vi "Load Macro.vi"(7 "Macro Name":string, 8 "error in (no error)":errorcluster, 11 "refnum":T5) -> (0 "error out":errorcluster, 2 "Macro":T1, 3 "refnum out":T5)   [LabVIEW 2020, in "MacroAssert.lvlib"]
doc: "Loads the macro defined by <B>Macro Name</B> from the config file defined by <B>refnum</B>."
uses:
  MacroAssert.lvlib
  <vilib>/Utility/config.llb/Config Data RefNum.ctl
  CTLs/Macro Cluster V3.ctl
  CTLs/Macro Config V3.ctl
  CTLs/Step V3.ctl
  CTLs/Step Type V3.ctl
  CTLs/Macro Cluster V1.ctl
  CTLs/Step V1-2.ctl
  CTLs/Step Type V1-2.ctl
  CTLs/Macro Cluster V2.ctl
  <vilib>/Utility/config.llb/Read Key (String).vi
  <vilib>/Utility/config.llb/Read Key (U32).vi
  <vilib>/Utility/config.llb/Read Key (I32).vi
  <vilib>/Utility/error.llb/Error Cluster From Error Code.vi
  <vilib>/ErrorRing/Error Ring.xnode
  <vilib>/Utility/config.llb/NI_LVConfig.lvlib
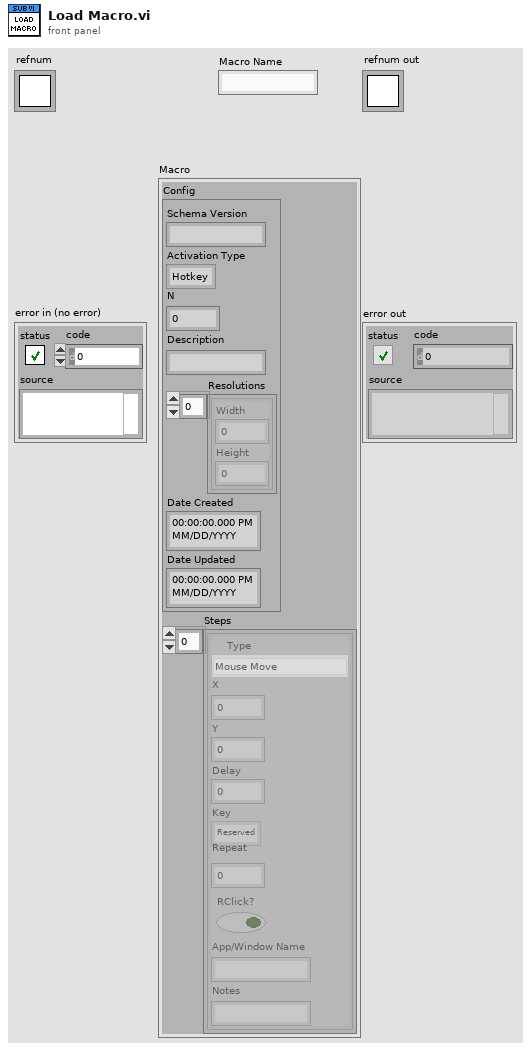
[diagram p1: front panel]
types:
  T1 = typedef "MacroAssert.lvlib/Macro Cluster V3.ctl" = cluster{"Config":T2, "Steps":T3[]}
  T2 = typedef "MacroAssert.lvlib/Macro Config V3.ctl" = cluster{"Schema Version":string, "Activation Type":enum32{"Hotkey", "Automatic"}, "N":i32, "Description":string, "Resolutions":cluster{"Width":i16, "Height":i16}[], "Date Created":timestamp, "Date Updated":timestamp}
  T3 = typedef "MacroAssert.lvlib/Step V3.ctl" = cluster{"Type":T4, "X":i32, "Y":i32, "Delay":i32, "Key":u8, "Repeat":i32, "RClick?":bool, "App/Window Name":string, "Notes":string}
  T4 = typedef "MacroAssert.lvlib/Step Type V3.ctl" = enum16{"Mouse Move", "Mouse Click", "Key Press", "Wait", "Mouse Down", "Mouse Up", "Key Down", "Key Up", "Run Application", "Maximize Window", "Restore Window", "Minimize Window", "Close Window", "Bring Window to Front", "Send Window to Back"}
  T5 = typedef "NI_LVConfig.lvlib/Config Data RefNum.ctl" = refnum<k1>
  T6 = typedef "MacroAssert.lvlib/Macro Cluster V1.ctl" = cluster{"Steps":T7[], "Activation Type":enum32{"Hotkey", "Automatic"}, "N":i32}
  T7 = typedef "MacroAssert.lvlib/Step V1-2.ctl" = cluster{"Type":T8, "Coords":cluster{"x":i32, "y":i32}, "Delay":i32, "Key":u8, "Repeat":i32, "RClick?":bool}
  T8 = typedef "MacroAssert.lvlib/Step Type V1-2.ctl" = enum16{"Mouse Move", "Mouse Click", "Key Press", "Wait", "Mouse Down", "Mouse Up", "Key Down", "Key Up"}
  T9 = typedef "MacroAssert.lvlib/Macro Cluster V2.ctl" = cluster{"Steps":T7[], "Activation Type":enum32{"Hotkey", "Automatic"}, "N":i32, "Description":string, "Resolutions":cluster{"Width":i16, "Height":i16}[], "Date Created":timestamp, "Date Updated":timestamp}
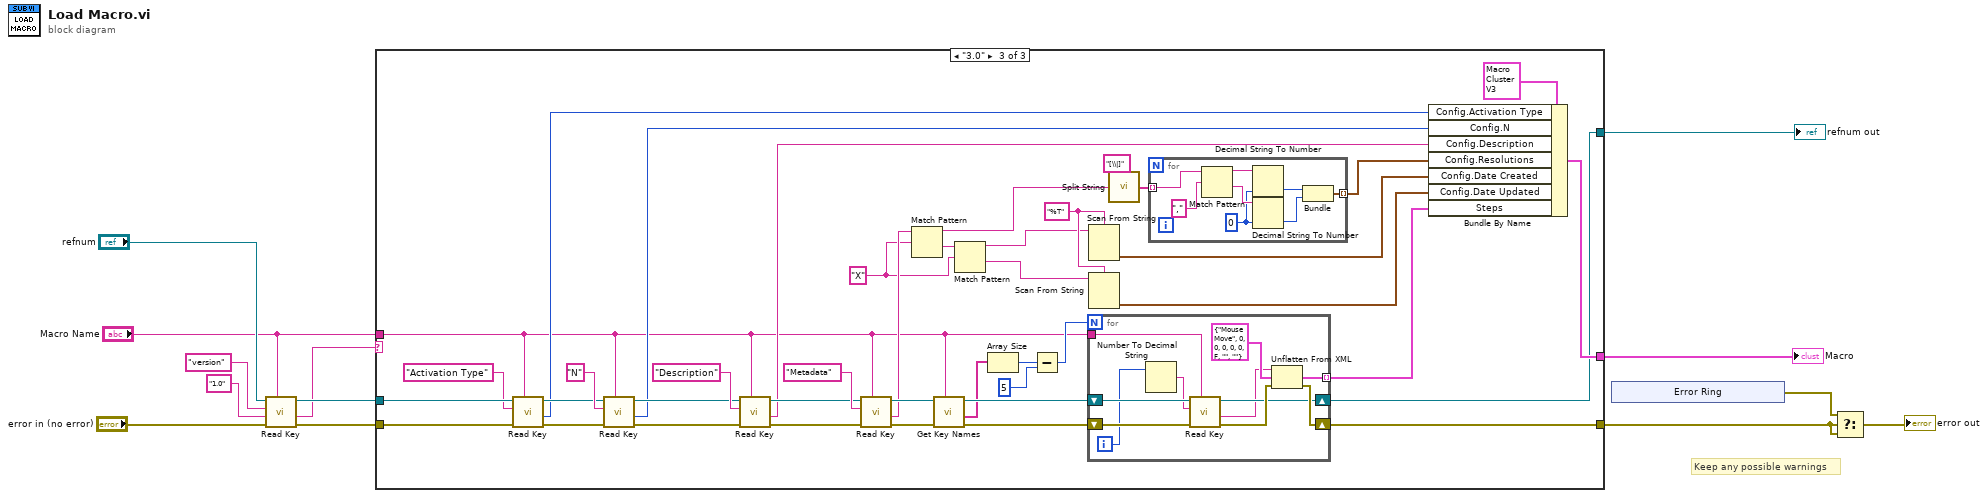
[diagram p0: block diagram]
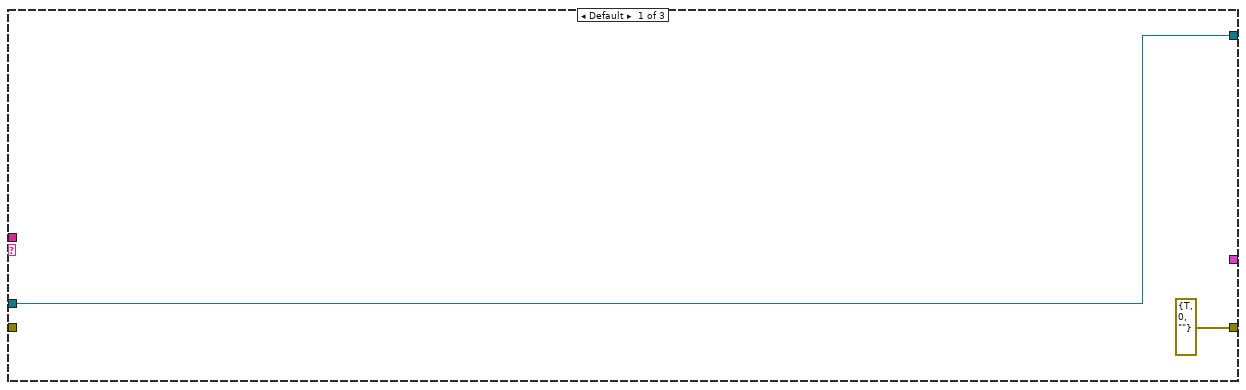
[diagram p2: hidden frame]
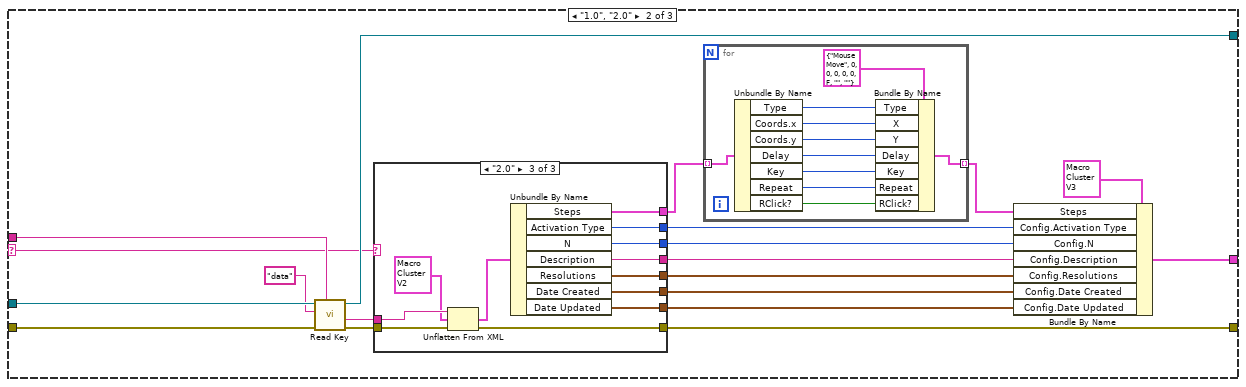
[diagram p3: hidden frame]
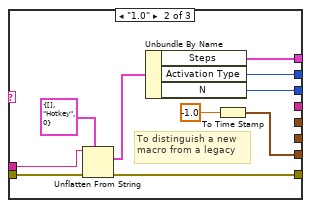
[diagram p5: hidden frame]
diagram:
  # "Keep any possible warnings"
  n1 = call-poly <vilib>:"Read Key.vi"("section"="Macro Name", "error in (no error)"="error in (no error)", "default value"="1.0", "key"="version", "refnum"="refnum") -> ("error out"=w9:errorcluster, "value"=w5:string, "refnum out"=w12:T5)  [unwired: 3 in, 1 out]
  n2 = case shown="\"3.0\"" w5 {
    selector: w5 -> [_ w27 _]
    tunnel: w12 -> [w15 w34 w108]
    tunnel: [w15 w30 w75] -> w11
    tunnel: w9 -> [_ w29 w106]
    tunnel: "Macro Name" -> [_ w28 w68]
    tunnel: [errorcluster {"status"=TRUE, "code"=0, "source"=""} ("error out") w20 w88] -> w3
    tunnel: [_ w19 w105] -> w4
    frame Default {
    }
    frame "1.0", "2.0" {
      n3 = call-poly <vilib>:"Read Key.vi"("section"=w28, "error in (no error)"=w29, "key"="data", "refnum"=w34) -> ("error out"=w31:errorcluster, "value"=w32:string, "refnum out"=w30:T5)  [unwired: 4 in, 1 out]
      n4 = case shown="\"2.0\"" w27 {
        tunnel: w32 -> [_ w55 w67]
        tunnel: w31 -> [w45 w54 w66]
        tunnel: [w45 w53 w65] -> w20
        tunnel: [_ w51 w63] -> w17
        tunnel: [_ w50 w62] -> w26
        tunnel: [_ w49 w61] -> w25
        tunnel: [_ _ w59] -> w24
        tunnel: [_ _ w58] -> w23
        tunnel: [_ _ w57] -> w22
        tunnel: [_ w46 w56] -> w21
        frame "False", Default {
        }
        frame "1.0" {
          # "To distinguish a new macro from a legacy"
          n5 = Unflatten From String(type=T6 {"Steps"=[], "Activation Type"=enum."Hotkey", "N"=0} ("Macro Cluster"), binary string=w55, error in (no error)=w54) -> (value=w52:T6, error out=w53:errorcluster)  [unwired: 2 in, 1 out]
          n6 = Unbundle By Name(w52) -> ("Steps"=w51:T7[], "Activation Type"=w50:enum32{"Hotkey", "Automatic"}, "N"=w49:i32)
          n7 = To Time Stamp(1:-1.0) -> (0:w46:timestamp)
        }
        frame "2.0" {
          n8 = Unflatten From XML(xml string=w67, type=T9 {"Steps"=[], "Activation Type"=enum."Hotkey", "N"=0, "Description"="", "Resolutions"=[], "Date Created"=timestamp(0 s since 1904-01-01), "Date Updated"=timestamp(0 s since 1904-01-01)} ("Macro Cluster"), error in (no error)=w66) -> (value=w64:T9, error out=w65:errorcluster)
          n9 = Unbundle By Name(w64) -> ("Steps"=w63:T7[], "Activation Type"=w62:enum32{"Hotkey", "Automatic"}, "N"=w61:i32, "Description"=w59:string, "Resolutions"=w58:cluster{"Width":i16, "Height":i16}[], "Date Created"=w57:timestamp, "Date Updated"=w56:timestamp)
        }
      }
      n10 = for {
        tunnel: w17 -> [w44] mode=indexing
        tunnel: [w37] -> w16 mode=indexing
        n11 = Unbundle By Name(w44) -> ("Type"=w36:T8, "Coords.x"=w42:i32, "Coords.y"=w35:i32, "Delay"=w41:i32, "Key"=w40:u8, "Repeat"=w39:i32, "RClick?"=w38:bool)
        n12 = Bundle By Name(cluster=T3 {"Type"=enum."Mouse Move", "X"=0, "Y"=0, "Delay"=0, "Key"=0, "Repeat"=0, "RClick?"=FALSE, "App/Window Name"="", "Notes"=""} ("Step"), "Type"=w36, "X"=w42, "Y"=w35, "Delay"=w41, "Key"=w40, "Repeat"=w39, "RClick?"=w38) -> (w37:T3)
      }
      n13 = Bundle By Name(cluster=T1 {"Config"={"Schema Version"="", "Activation Type"=enum."Hotkey", "N"=0, "Description"="", "Resolutions"=[], "Date Created"=timestamp(0 s since 1904-01-01), "Date Updated"=timestamp(0 s since 1904-01-01)}, "Steps"=[]} ("Macro Cluster"), "Steps"=w16, "Config.Activation Type"=w26, "Config.N"=w25, "Config.Description"=w24, "Config.Resolutions"=w23, "Config.Date Created"=w22, "Config.Date Updated"=w21) -> (w19:T1)
    }
    frame "3.0" {
      w72 = "X" ("Split Pattern")
      w91 = "%T" ("format string")
      n14 = call-poly <vilib>:"Read Key.vi"("section"=w68, "error in (no error)"=w106, "key"="Activation Type", "refnum"=w108) -> ("error out"=w101:errorcluster, "value"=w94:u32, "refnum out"=w102:T5)  [unwired: 4 in, 1 out]
      n15 = call-poly <vilib>:"Read Key.vi"("section"=w68, "error in (no error)"=w101, "key"="N", "refnum"=w102) -> ("error out"=w98:errorcluster, "value"=w93:i32, "refnum out"=w99:T5)  [unwired: 4 in, 1 out]
      n16 = call-poly <vilib>:"Read Key.vi"("section"=w68, "error in (no error)"=w98, "key"="Description", "refnum"=w99) -> ("error out"=w95:errorcluster, "value"=w92:string, "refnum out"=w96:T5)  [unwired: 4 in, 1 out]
      n17 = call-poly <vilib>:"Read Key.vi"("section"=w68, "error in (no error)"=w95, "key"="Metadata", "refnum"=w96) -> ("error out"=w83:errorcluster, "value"=w74:string, "refnum out"=w82:T5)  [unwired: 4 in, 1 out]
      n18 = Match Pattern(string=w74, regular expression=w72) -> (before substring=w71:string, after substring=w73:string)  [unwired: 1 in, 2 out]
      n19 = call <vilib>:"Get Key Names.vi"("section"=w68, "error in (no error)"=w83, "refnum"=w82) -> ("error out"=w81:errorcluster, "key names"=w79:string[], "refnum out"=w80:T5)  [unwired: 5 in, 1 out]
      n20 = Match Pattern(string=w73, regular expression=w72) -> (before substring=w70:string, after substring=w69:string)  [unwired: 1 in, 2 out]
      n21 = Array Size(array=w79) -> (size(s)=w78:i32)
      n22 = Subtract(x=w78, y=5) -> (x-y=w76:i32)
      n23 = for {
        N: w76 -> [_]
        tunnel: [w125] -> w87 mode=indexing
        shift-right: [w126] -> w88
        shift-left: w81 -> [w121]
        shift-right: [w122] -> w75
        shift-left: w80 -> [w124]
        tunnel: w68 -> [w120]
        i -> [w118]
        n24 = Number To Decimal String(number=w118) -> (decimal integer string=w119:string)  [unwired: 1 in]
        n25 = call-poly <vilib>:"Read Key.vi"("section"=w120, "error in (no error)"=w121, "key"=w119, "refnum"=w124) -> ("error out"=w123:errorcluster, "value"=w117:string, "refnum out"=w122:T5)  [unwired: 4 in, 1 out]
        n26 = Unflatten From XML(xml string=w117, type=T3 {"Type"=enum."Mouse Move", "X"=0, "Y"=0, "Delay"=0, "Key"=0, "Repeat"=0, "RClick?"=FALSE, "App/Window Name"="", "Notes"=""} ("Step"), error in (no error)=w123) -> (value=w125:T3, error out=w126:errorcluster)
      }
      n27 = Scan From String(format string=w91, input string=w70) -> (output 1=w90:timestamp)  [unwired: 3 in, 3 out]
      n28 = Scan From String(format string=w91, input string=w69) -> (output 1=w89:timestamp)  [unwired: 3 in, 3 out]
      n29 = call <vilib>:"Split String.vi"("Split Pattern"="[\\|]", "Input String"=w71) -> ("Split String"=w85:string[])  [unwired: 5 in]
      n30 = for {
        tunnel: w85 -> [w116] mode=indexing
        tunnel: [w110] -> w84 mode=indexing
        w109 = i16 0 ("default (0 I32)")
        n31 = Match Pattern(string=w116, regular expression=",") -> (before substring=w114:string, after substring=w113:string)  [unwired: 1 in, 2 out]
        n32 = Decimal String To Number(string=w114, default (0L)=w109) -> (number=w112:i16)  [unwired: 1 in, 1 out]
        n33 = Decimal String To Number(string=w113, default (0L)=w109) -> (number=w111:i16)  [unwired: 1 in, 1 out]
        n34 = Bundle(w112, w111) -> (w110:cluster{i16, i16})  [unwired: 1 in]
      }
      n35 = Bundle By Name(cluster=T1 {"Config"={"Schema Version"="", "Activation Type"=enum."Hotkey", "N"=0, "Description"="", "Resolutions"=[], "Date Created"=timestamp(0 s since 1904-01-01), "Date Updated"=timestamp(0 s since 1904-01-01)}, "Steps"=[]} ("Macro Cluster"), "Config.Activation Type"=w94, "Config.N"=w93, "Config.Description"=w92, "Config.Resolutions"=w84, "Config.Date Created"=w90, "Config.Date Updated"=w89, "Steps"=w87) -> (w105:T1)
    }
  }
  "refnum out" <- w11
  "Macro" <- w4
  n36 = xnode "Error Ring"() -> ("error out"=w2:errorcluster)
  n37 = Select(t=w2, s=w3, f=w3) -> (s? t:f=→"error out":errorcluster)
